vi "backward difference system.vi"(1 "Input sequence x[n]":dbl[](array[numeric])=[1.0, 2.0, 3.0]) -> (0 "B[n] = x[n] - x[n-1]":dbl[](array[numeric])=[1.0, 1.0, 1.0] format="%#.0f")   [LabVIEW 2009]
uses:
  <vilib>/Analysis/2dsp.llb/1D Convolution (DBL).vi
  <vilib>/Analysis/NI_AALBase.lvlib
  <vilib>/Analysis/NI_AALPro.lvlib
panel:
  out "B[n] = x[n] - x[n-1]":dbl[](graph)=[1.0, 1.0, 1.0]
  out "initialized array":dbl[](array[numeric])
  out "Input Sequence x[n]":dbl[](graph)=[1.0, 2.0, 3.0]
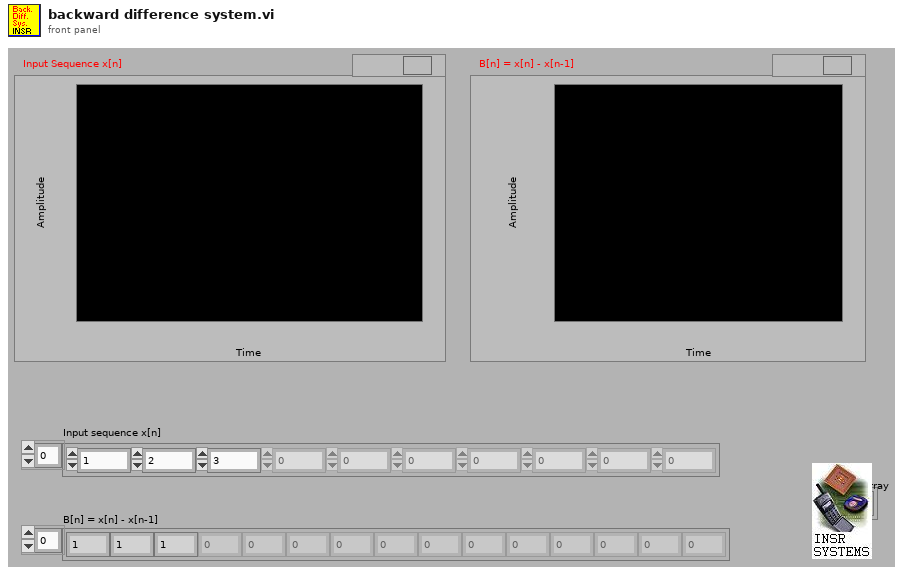
[diagram p1: front panel]
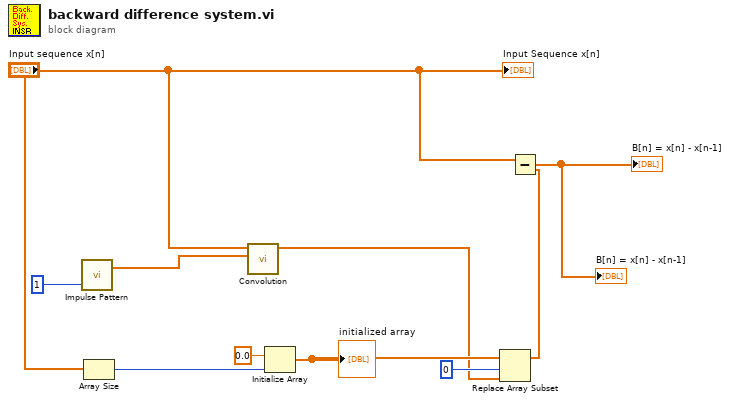
[diagram p0: block diagram]
diagram:
  n1 = call <vilib>:"Impulse Pattern.vi"("delay"=1) -> ("Impulse Pattern"=w10:dbl[])  [unwired: 2 in, 1 out]
  n2 = Array Size(array="Input sequence x[n]") -> (size(s)=w8:i32)
  n3 = call-poly <vilib>:"Convolution.vi"("Y"=w10, "X"="Input sequence x[n]") -> ("X * Y"=w4:dbl[])  [unwired: 8 in, 1 out]
  n4 = Initialize Array(0.0 ("element"), w8) -> (w6:dbl[])
  "initialized array" <- w6
  n5 = Replace Array Subset(array=w6, new element=w4, index=0) -> (w2:dbl[])
  n6 = Subtract(x="Input sequence x[n]", y=w2) -> (x-y=→"B[n] = x[n] - x[n-1]" →"B[n] = x[n] - x[n-1]":dbl[])
  "Input Sequence x[n]" <- "Input sequence x[n]"
